vi "Data - relative_file_path_handling.vi"(8 "error in":errorcluster, 11 "path in":path) -> (0 "error out":errorcluster, 3 "path out":path)   [LabVIEW 2019]
doc: "This is the general vi used to strip input file path to get the folder path that leads to that component based upon the type of enviroment the VI is running in\n1. LabVIEW development enviroment\n\n2. stand-alone application\n\nChenny Wang\n01/09/2007"
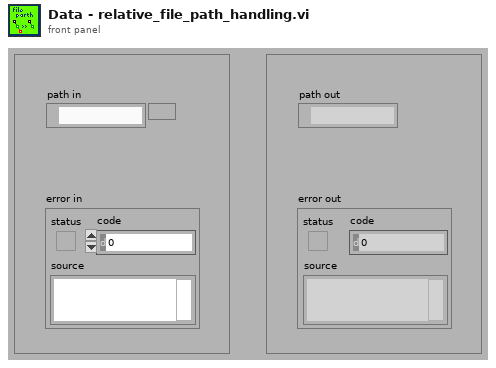
[diagram p1: front panel]
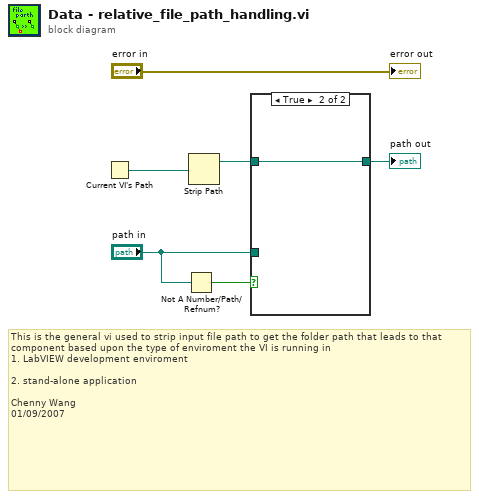
[diagram p0: block diagram]
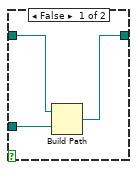
[diagram p2: hidden frame]
diagram:
  # "This is the general vi used to strip input file path to get the folder path that leads to that component based upon the type of enviroment the VI is running in\n1. LabVIEW development enviroment\n\n2. stand-alone application\n\nChenny Wang\n01/09/2007"
  n1 = Current VI's Path() -> (path=w6:path)
  n2 = Not A Number/Path/Refnum?(number/path/refnum="path in") -> (NaN/Path/Refnum?=w5:bool)
  n3 = Strip Path(path=w6) -> (stripped path=w2:path)  [unwired: 1 out]
  n4 = case shown="True" w5 {
    tunnel: w2 -> [w9 w10]
    tunnel: "path in" -> [w8 _]
    tunnel: [w7 w10] -> w3
    frame False {
      n5 = Build Path(base path=w9, name or relative path=w8) -> (appended path=w7:path)
    }
    frame True {
    }
  }
  "path out" <- w3
  "error out" <- "error in"
